vi "Start Instruments.vi"(8 "Error In":errorcluster, 11 "reference in":refnum<class "Measure and Stimulus Subsystems.lvclass">) -> (0 "Error Out":errorcluster, 3 "reference out":refnum<class "Measure and Stimulus Subsystems.lvclass">)   [LabVIEW 2023, in "HAL GOOP4.lvlib" / "Measure and Stimulus Subsystems.lvclass"]
uses:
  Measure and Stimulus Subsystems.lvclass
  Instrument/Instrument.lvclass
  Measure and Stimulus Subsystems.lvclass/Measure and Stimulus Subsystems.ctl
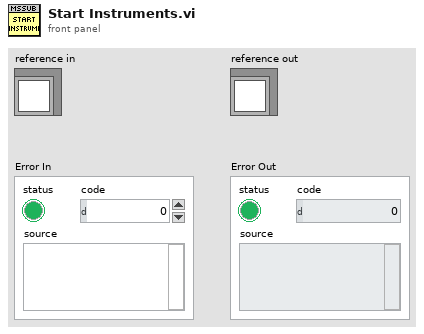
[diagram p1: front panel]
types:
  T1 = typedef "HAL GOOP4.lvlib/Measure and Stimulus Subsystems.lvclass/ObjectAttributes.ctl" = cluster{"Virt Instr":map{string, refnum<class "Virt Instr Base.lvclass">}, "Phys Instr":map{string, cluster{"Instrument Base":refnum<class "Instrument.lvclass">, "Ref Count":u8}}}
  T2 = map{string, cluster{"Instrument Base":refnum<class "Instrument.lvclass">, "Ref Count":u8}}
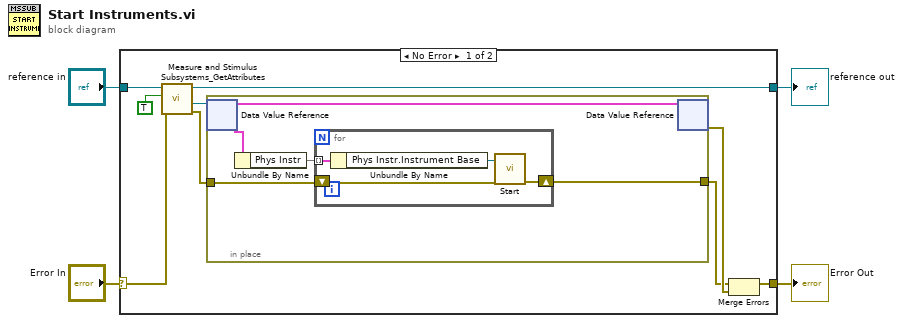
[diagram p0: block diagram]
diagram:
  n1 = case shown="No Error" "Error In" {
    selector: "Error In" -> [w12 w23]
    tunnel: [w9 w23] -> w3
    tunnel: [w10 w22] -> w1
    tunnel: "reference in" -> [w13 w22]
    frame No Error {
      n2 = call "Measure and Stimulus Subsystems_GetAttributes.vi"("Error In"=w12, "OnlyGetDvrReference(False)"=TRUE, "reference in"=w13) -> ("Error Out"=w6:errorcluster, "DataRef"=w8:refnum<data-value>, "reference out"=w10:refnum<class "Measure and Stimulus Subsystems.lvclass">)  [unwired: 5 in, 1 out]
      n3 = in-place {
        in-place-border: w6 -> [w16]
        in-place-border: [w14] -> w5
        n4 = in-place-dvr #1(w8) -> (w15:T1)  [unwired: 1 out]
        n5 = Unbundle By Name(w15) -> ("Phys Instr"=w17:T2)
        n6 = for {
          tunnel: w17 -> [w21] mode=indexing
          shift-right: [w18] -> w14
          shift-left: w16 -> [w19]
          n7 = Unbundle By Name(w21) -> ("Phys Instr.Instrument Base"=w20:refnum<class "Instrument.lvclass">)
          n8 = call-dynamic "Start.vi"("error in (no error)"=w19, "reference in"=w20) -> ("error out"=w18:errorcluster)  [unwired: 8 in, 1 out]
        }
        n9 = in-place-dvr #1(w15) -> (w11:errorcluster)  [unwired: 1 out]
      }
      n10 = Merge Errors(w5, w11) -> (w9:errorcluster)
    }
    frame Error {
    }
  }
  "Error Out" <- w3
  "reference out" <- w1
